vi "TruthTable7seg.vi"(1 "task/channels in":refnum<k21>, 2 "Numeric Control":i32) -> (0 "error out 2":errorcluster)   [LabVIEW 2015]
doc: "This VI control a 7-segment display, \n\nInput | 7 segment display Output\n0 , 0\n1, 1\n2, 2\n3, 3\n4, 4\n5, 5\n6, 6\n7, 7\n8, 8\n9, 9\n10, .\n11, OFF"
uses:
  <vilib>/DAQmx/write.llb/DAQmx Write (Digital 1D Bool 1Chan 1Samp).vi
  <vilib>/DAQmx/miscellaneous.llb/DAQmx Fill In Error Info.vi
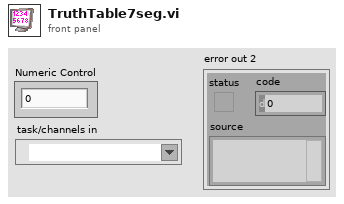
[diagram p1: front panel]
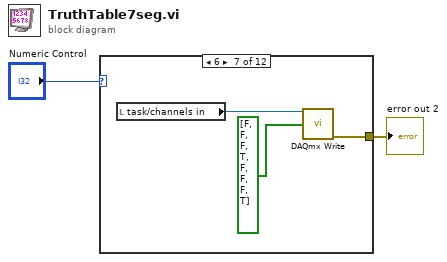
[diagram p0: block diagram]
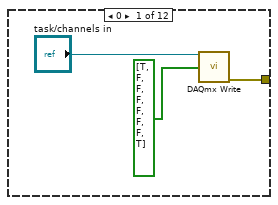
[diagram p2: hidden frame]
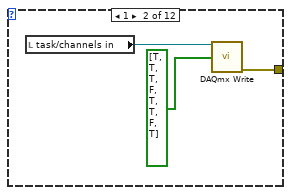
[diagram p3: hidden frame]
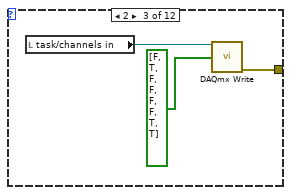
[diagram p4: hidden frame]
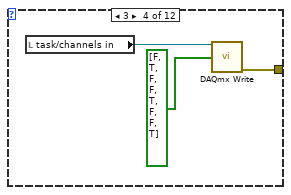
[diagram p5: hidden frame]
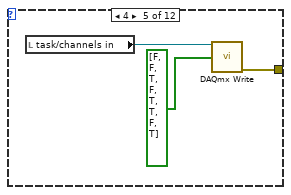
[diagram p6: hidden frame]
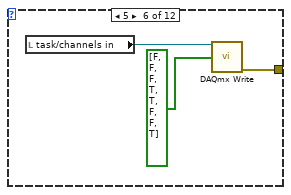
[diagram p7: hidden frame]
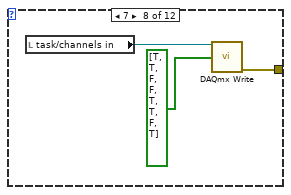
[diagram p8: hidden frame]
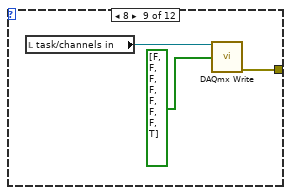
[diagram p9: hidden frame]
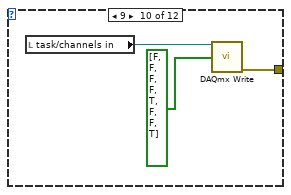
[diagram p10: hidden frame]
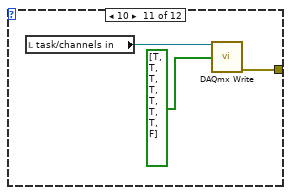
[diagram p11: hidden frame]
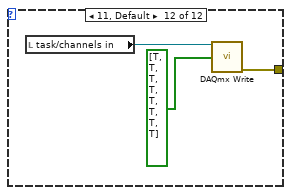
[diagram p12: hidden frame]
diagram:
  n1 = case shown="6" "Numeric Control" {
    tunnel: [w3 w6 w9 w12 w15 w18 w21 w24 w27 w30 w33 w37] -> w2
    frame 0 {
      n2 = call-poly <vilib>:"DAQmx Write.vi"("task/channels in"="task/channels in", "data"=bool[] [TRUE, FALSE, FALSE, FALSE, FALSE, FALSE, FALSE, TRUE]) -> ("error out"=w3:errorcluster)  [unwired: 11 in, 2 out]
    }
    frame 1 {
      n3 = local read "task/channels in"() -> (w8:refnum<k21>)
      n4 = call-poly <vilib>:"DAQmx Write.vi"("task/channels in"=w8, "data"=bool[] [TRUE, TRUE, TRUE, FALSE, TRUE, TRUE, FALSE, TRUE] ("data 2")) -> ("error out"=w6:errorcluster)  [unwired: 11 in, 2 out]
    }
    frame 2 {
      n5 = local read "task/channels in"() -> (w10:refnum<k21>)
      n6 = call-poly <vilib>:"DAQmx Write.vi"("task/channels in"=w10, "data"=bool[] [FALSE, TRUE, FALSE, FALSE, FALSE, FALSE, TRUE, TRUE] ("data 3")) -> ("error out"=w9:errorcluster)  [unwired: 11 in, 2 out]
    }
    frame 3 {
      n7 = local read "task/channels in"() -> (w13:refnum<k21>)
      n8 = call-poly <vilib>:"DAQmx Write.vi"("task/channels in"=w13, "data"=bool[] [FALSE, TRUE, FALSE, FALSE, TRUE, FALSE, FALSE, TRUE] ("data 4")) -> ("error out"=w12:errorcluster)  [unwired: 11 in, 2 out]
    }
    frame 4 {
      n9 = local read "task/channels in"() -> (w16:refnum<k21>)
      n10 = call-poly <vilib>:"DAQmx Write.vi"("task/channels in"=w16, "data"=bool[] [FALSE, FALSE, TRUE, FALSE, TRUE, TRUE, FALSE, TRUE] ("data 5")) -> ("error out"=w15:errorcluster)  [unwired: 11 in, 2 out]
    }
    frame 5 {
      n11 = local read "task/channels in"() -> (w19:refnum<k21>)
      n12 = call-poly <vilib>:"DAQmx Write.vi"("task/channels in"=w19, "data"=bool[] [FALSE, FALSE, FALSE, TRUE, TRUE, FALSE, FALSE, TRUE] ("data 6")) -> ("error out"=w18:errorcluster)  [unwired: 11 in, 2 out]
    }
    frame 6 {
      n13 = local read "task/channels in"() -> (w22:refnum<k21>)
      n14 = call-poly <vilib>:"DAQmx Write.vi"("task/channels in"=w22, "data"=bool[] [FALSE, FALSE, FALSE, TRUE, FALSE, FALSE, FALSE, TRUE] ("data 7")) -> ("error out"=w21:errorcluster)  [unwired: 11 in, 2 out]
    }
    frame 7 {
      n15 = local read "task/channels in"() -> (w25:refnum<k21>)
      n16 = call-poly <vilib>:"DAQmx Write.vi"("task/channels in"=w25, "data"=bool[] [TRUE, TRUE, FALSE, FALSE, TRUE, TRUE, FALSE, TRUE] ("data 8")) -> ("error out"=w24:errorcluster)  [unwired: 11 in, 2 out]
    }
    frame 8 {
      n17 = local read "task/channels in"() -> (w28:refnum<k21>)
      n18 = call-poly <vilib>:"DAQmx Write.vi"("task/channels in"=w28, "data"=bool[] [FALSE, FALSE, FALSE, FALSE, FALSE, FALSE, FALSE, TRUE] ("data 9")) -> ("error out"=w27:errorcluster)  [unwired: 11 in, 2 out]
    }
    frame 9 {
      n19 = local read "task/channels in"() -> (w31:refnum<k21>)
      n20 = call-poly <vilib>:"DAQmx Write.vi"("task/channels in"=w31, "data"=bool[] [FALSE, FALSE, FALSE, FALSE, TRUE, FALSE, FALSE, TRUE] ("data 10")) -> ("error out"=w30:errorcluster)  [unwired: 11 in, 2 out]
    }
    frame 10 {
      n21 = local read "task/channels in"() -> (w34:refnum<k21>)
      n22 = call-poly <vilib>:"DAQmx Write.vi"("task/channels in"=w34, "data"=bool[] [TRUE, TRUE, TRUE, TRUE, TRUE, TRUE, TRUE, FALSE] ("data 11")) -> ("error out"=w33:errorcluster)  [unwired: 11 in, 2 out]
    }
    frame 11, Default {
      n23 = local read "task/channels in"() -> (w38:refnum<k21>)
      n24 = call-poly <vilib>:"DAQmx Write.vi"("task/channels in"=w38, "data"=bool[] [TRUE, TRUE, TRUE, TRUE, TRUE, TRUE, TRUE, TRUE]) -> ("error out"=w37:errorcluster)  [unwired: 11 in, 2 out]
    }
  }
  "error out 2" <- w2
